vi "trabajo23-12-20.vi"() -> ()   [LabVIEW 2020]
panel:
  out "AREA DEL TRIANGULO":dbl
  in  "ALTURA":dbl
  in  "BASE":dbl
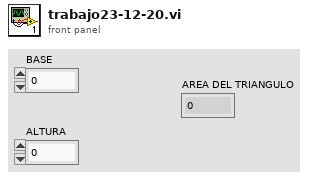
[diagram p1: front panel]
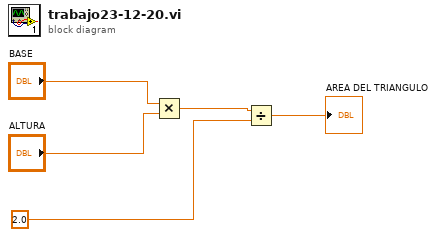
[diagram p0: block diagram]
diagram:
  n1 = Multiply(x="BASE", y="ALTURA") -> (x*y=w3:dbl)
  n2 = Divide(x=w3, y=2.0) -> (x/y=→"AREA DEL TRIANGULO":dbl)
